vi "CounterClock.vi"() -> (0 "Counter clock rate divided by prescaler":dbl=80000000.0, 1 "Counter clock rate":dbl=80000000.0, 2 "Clock division factor":dbl=1.0, 3 "CI.Prescaler":u32=1)   [LabVIEW 2018]
uses:
  global_channels.vi
panel:
  out "Prescaler":u16(ring) items=["1x", "2x", "8x"]
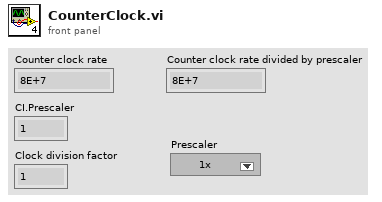
[diagram p1: front panel]
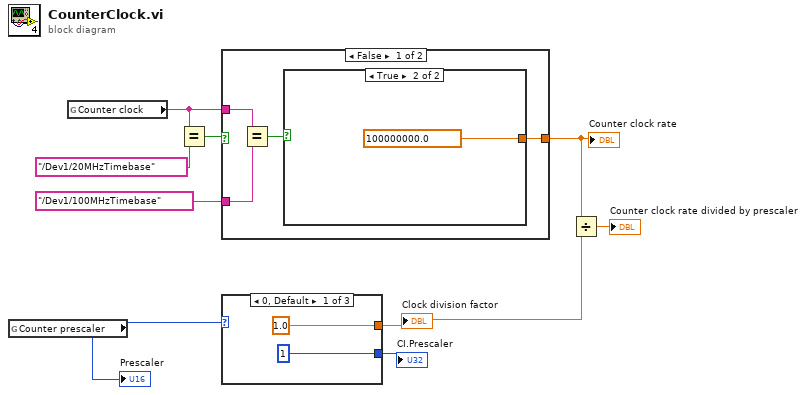
[diagram p0: block diagram]
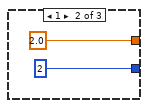
[diagram p2: hidden frame]
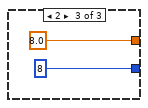
[diagram p3: hidden frame]
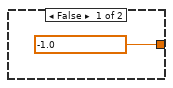
[diagram p4: hidden frame]
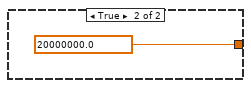
[diagram p5: hidden frame]
diagram:
  n1 = global read "global_channels.vi" "Counter prescaler"() -> (w3:u16)
  "Prescaler" <- w3
  n2 = global read "global_channels.vi" "Counter clock"() -> (w6:tag)
  n3 = Equal?(x=w6, y=tag "/Dev1/20MHzTimebase" ("Counter clock")) -> (x = y?=w9:bool)
  n4 = case shown="False" w9 {
    tunnel: tag "/Dev1/100MHzTimebase" ("Counter clock") -> [w13 _]
    tunnel: w6 -> [w12 _]
    tunnel: [w10 20000000.0 ("Counter clock rate")] -> w5
    frame False {
      n5 = Equal?(x=w12, y=w13) -> (x = y?=w11:bool)
      n6 = case shown="True" w11 {
        tunnel: [-1.0 ("Counter clock rate") 100000000.0 ("Counter clock rate")] -> w10
        frame False {
        }
        frame True {
        }
      }
    }
    frame True {
    }
  }
  "Counter clock rate" <- w5
  n7 = case shown="0, Default" w3 {
    tunnel: [1.0 ("y") 2.0 ("y") 8.0 ("y")] -> w1
    tunnel: [u32 1 ("CI.Prescaler") u32 2 ("CI.Prescaler") u32 8 ("CI.Prescaler")] -> w2
    frame 0, Default {
    }
    frame 1 {
    }
    frame 2 {
    }
  }
  "CI.Prescaler" <- w2
  "Clock division factor" <- w1
  n8 = Divide(x=w5, y=w1) -> (x/y=→"Counter clock rate divided by prescaler":dbl)
